vi "COD质控流程 (子VI).vi"(11 "COD":bool) -> (3 "布尔":bool)   [LabVIEW 2016, in "质控单元.lvlib"]
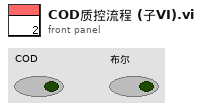
[diagram p1: front panel]
types:
  T1 = enum16{"待机", "启动水样测量", "水样测量中", "启动加标", "启动加标回收", "加标回收测量中", "结束"}
  T2 = cluster{"测量模式":enum16{"水样测量", "标样核查", "零点核查", "加标回收", "平行样", "校零", "校标"}}
  T3 = cluster{"量程":dbl, "检出限":dbl, "加标前水样浓度":dbl, "加标后水样浓度":dbl, "加标水杯定容体积":dbl, "加标母液浓度":dbl, "加标体积":dbl, "加标回收率":dbl}
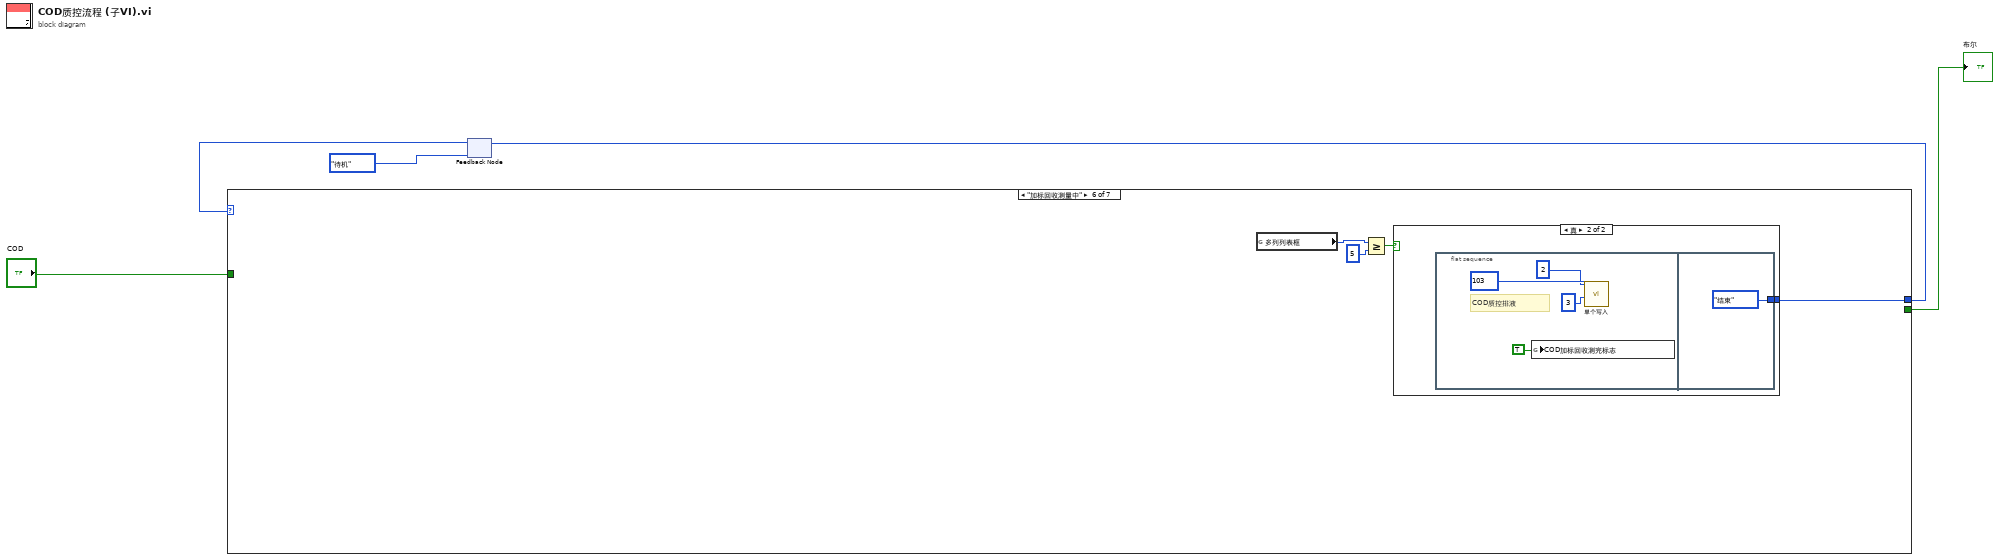
[diagram p0: block diagram]
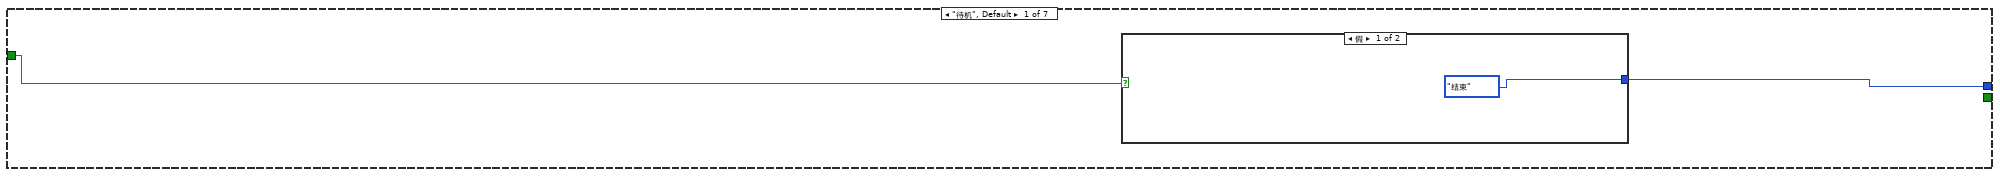
[diagram p2: hidden frame]
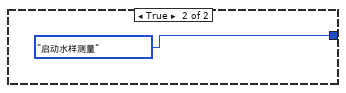
[diagram p3: hidden frame]
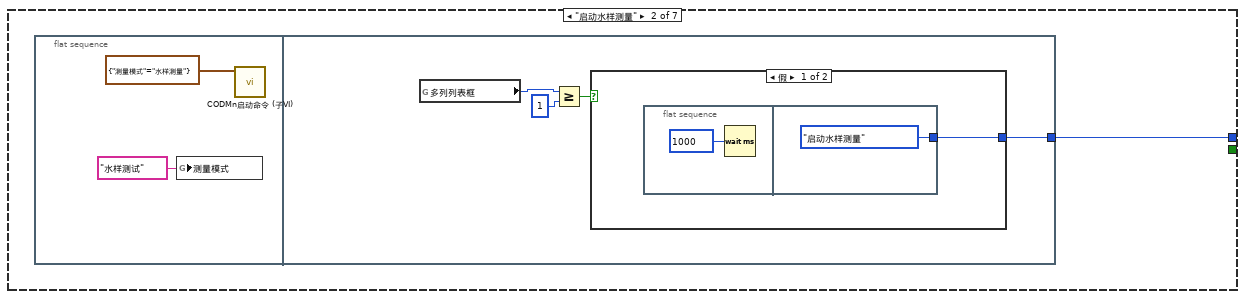
[diagram p4: hidden frame]
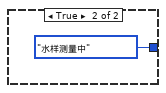
[diagram p5: hidden frame]
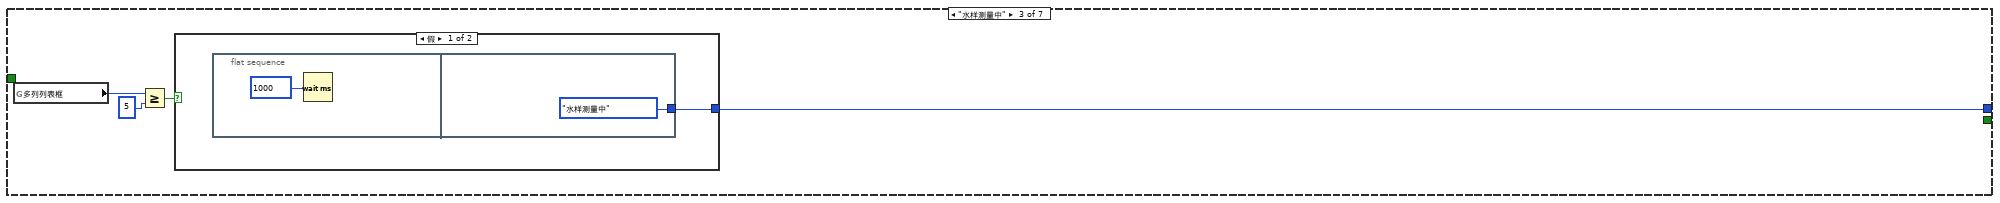
[diagram p6: hidden frame]
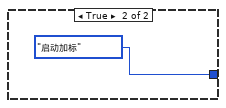
[diagram p7: hidden frame]
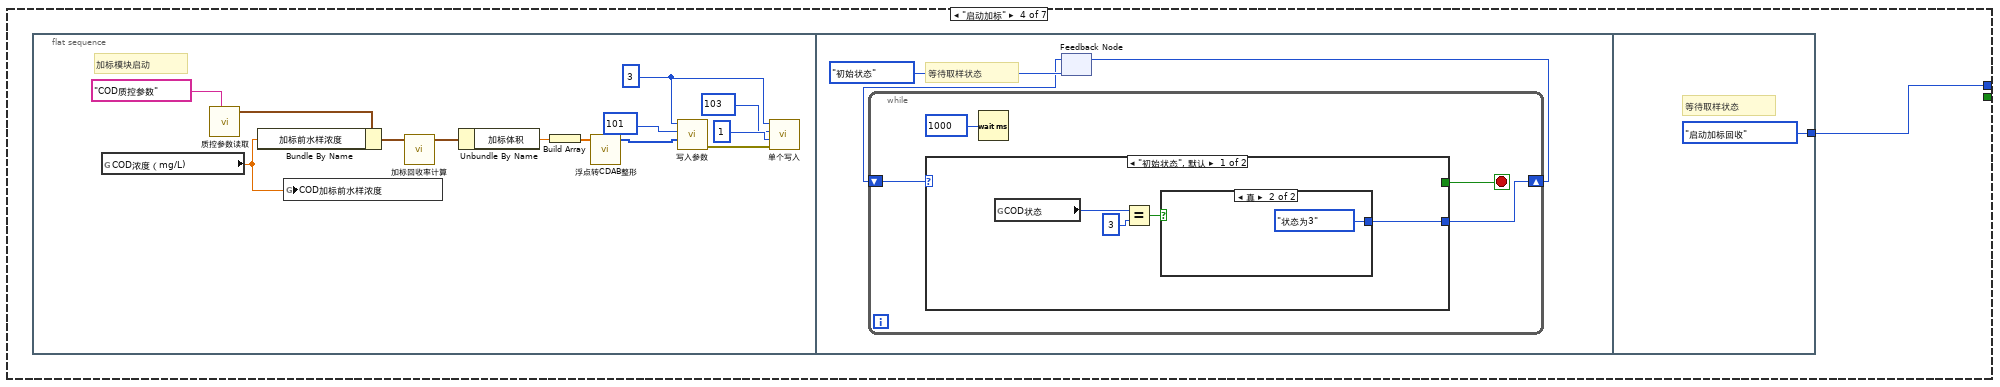
[diagram p8: hidden frame]
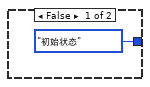
[diagram p9: hidden frame]
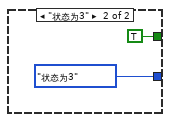
[diagram p10: hidden frame]
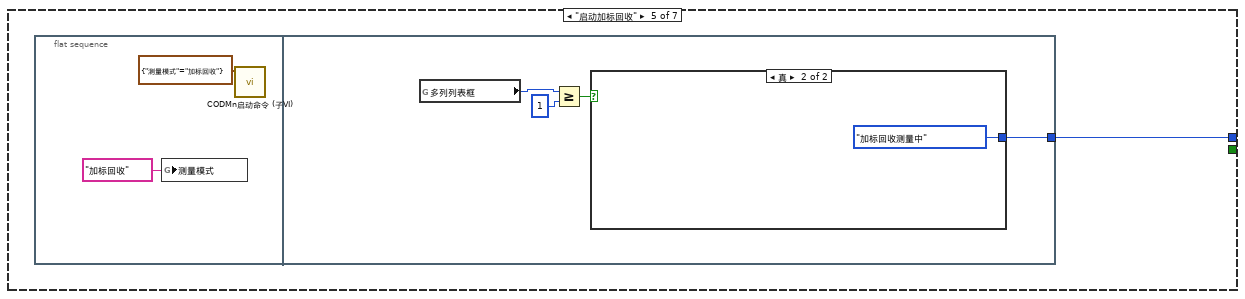
[diagram p11: hidden frame]
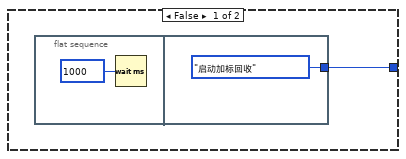
[diagram p12: hidden frame]
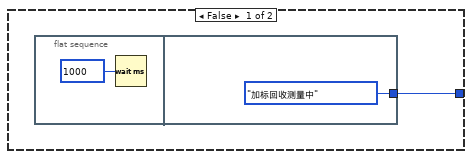
[diagram p13: hidden frame]
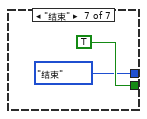
[diagram p14: hidden frame]
diagram:
  n1 = feedback #1(T1."待机") -> (w3:T1)
  n2 = case shown="\"加标回收测量中\"" w3 {
    tunnel: [w7 w10 w21 w29 w59 w70 T1."结束"] -> w4
    tunnel: [_ _ _ _ _ _ TRUE] -> w2
    tunnel: "COD" -> [w6 _ _ _ _ _ _]
    frame "待机", Default {
      n3 = case shown="假" w6 {
        tunnel: [T1."结束" T1."启动水样测量"] -> w7
        frame False {
        }
        frame True {
        }
      }
    }
    frame "启动水样测量" {
      n4 = flat-sequence {
        tunnel: [w13] -> w10
        frame #0 {
          n5 = global write "COD测量模式全局.vi" "测量模式"("水样测试" ("测量模式")) -> ()
          n6 = call "CODMn启动命令 (子VI).vi"("启动测量模式"=T2 {"测量模式"=enum."水样测量"}) -> ()  [unwired: 11 in]
        }
        frame #1 {
          n7 = global read "运行时序全局变量.vi" "多列列表框"() -> (w16:i32)
          n8 = Greater Or Equal?(x=w16, y=1) -> (x >= y?=w15:bool)
          n9 = case shown="假" w15 {
            tunnel: [w17 T1."水样测量中"] -> w13
            frame False {
              n10 = flat-sequence {
                tunnel: [T1."启动水样测量"] -> w17
                frame #0 {
                  n11 = Wait (ms)(milliseconds to wait=u32 1000 ("等待时间（毫秒）")) -> ()  [unwired: 1 out]
                }
                frame #1 {
                }
              }
            }
            frame True {
            }
          }
        }
      }
    }
    frame "水样测量中" {
      n12 = global read "运行时序全局变量.vi" "多列列表框"() -> (w22:i32)
      n13 = Greater Or Equal?(x=w22, y=5) -> (x >= y?=w23:bool)
      n14 = case shown="假" w23 {
        tunnel: [w25 T1."启动加标"] -> w21
        frame False {
          n15 = flat-sequence {
            tunnel: [T1."水样测量中"] -> w25
            frame #0 {
              n16 = Wait (ms)(milliseconds to wait=u32 1000 ("等待时间（毫秒）")) -> ()  [unwired: 1 out]
            }
            frame #1 {
            }
          }
        }
        frame True {
        }
      }
    }
    frame "启动加标" {
      n17 = flat-sequence {
        tunnel: [T1."启动加标回收"] -> w29
        frame #0 {
          w32 = u16 3 ("value")
          # "加标模块启动"
          n18 = global read "COD浓度全局变量.vi" "COD浓度（mg/L)"() -> (w30:dbl)
          n19 = call "质控参数读取.vi"("section"="COD质控参数") -> ("参数"=w40:T3)  [unwired: 9 in, 1 out]
          n20 = Bundle By Name(cluster=w40, "加标前水样浓度"=w30) -> (w41:T3)
          n21 = global write "水样浓度全局.vi" "COD加标前水样浓度"(w30) -> ()
          n22 = call "加标回收率计算.vi"("参数"=w41) -> ("参数 out"=w39:T3)  [unwired: 10 in]
          n23 = Unbundle By Name(w39) -> ("加标体积"=w31:dbl)
          n24 = Build Array(w31) -> (w38:dbl[])
          n25 = call "浮点转CDAB整形.vi"("浮点数"=w38) -> ("CDAB整形输出"=w33:u16[])  [unwired: 10 in]
          n26 = call "写入参数.vi"("values"=w33, "starting address"=u16 101, "Slave ID"=w32) -> ("error out"=w37:errorcluster)  [unwired: 8 in]
          n27 = call "单个写入.vi"("Error in"=w37, "value"=u16 1, "address"=u16 103, "Slave ID"=w32) -> ()  [unwired: 7 in, 1 out]
        }
        frame #1 {
          # "等待取样状态"
          n28 = feedback #2(enum16{"初始状态", "状态为3"}."初始状态") -> (w44:enum16{"初始状态", "状态为3"})
          n29 = while {
            shift-right: [w48] -> w43
            shift-left: w44 -> [w49]
            stop <- w47 stop-if-true
            n30 = case shown="\"初始状态\", 默认" w49 {
              tunnel: [w50 enum16{"初始状态", "状态为3"}."状态为3"] -> w48
              tunnel: [_ TRUE] -> w47
              frame "初始状态", Default {
                n31 = global read "氨氮加标回收状态全局变量.vi" "COD状态"() -> (w52:u16)
                n32 = Equal?(x=w52, y=u16 3) -> (x = y?=w51:bool)
                n33 = case shown="真" w51 {
                  tunnel: [enum16{"初始状态", "状态为3"}."初始状态" enum16{"初始状态", "状态为3"}."状态为3"] -> w50
                  frame False {
                  }
                  frame True {
                  }
                }
              }
              frame "状态为3" {
              }
            }
            n34 = Wait (ms)(milliseconds to wait=u32 1000 ("等待时间（毫秒）")) -> ()  [unwired: 1 out]
          }
          n35 = feedback-in #2(w43) -> ()
        }
        frame #2 {
          # "等待取样状态"
        }
      }
    }
    frame "启动加标回收" {
      n36 = flat-sequence {
        tunnel: [w62] -> w59
        frame #0 {
          n37 = global write "COD测量模式全局.vi" "测量模式"("加标回收" ("测量模式")) -> ()
          n38 = call "CODMn启动命令 (子VI).vi"("启动测量模式"=T2 {"测量模式"=enum."加标回收"}) -> ()  [unwired: 11 in]
        }
        frame #1 {
          n39 = global read "运行时序全局变量.vi" "多列列表框"() -> (w63:i32)
          n40 = Greater Or Equal?(x=w63, y=1) -> (x >= y?=w64:bool)
          n41 = case shown="真" w64 {
            tunnel: [w66 T1."加标回收测量中"] -> w62
            frame False {
              n42 = flat-sequence {
                tunnel: [T1."启动加标回收"] -> w66
                frame #0 {
                  n43 = Wait (ms)(milliseconds to wait=u32 1000 ("等待时间（毫秒）")) -> ()  [unwired: 1 out]
                }
                frame #1 {
                }
              }
            }
            frame True {
            }
          }
        }
      }
    }
    frame "加标回收测量中" {
      n44 = global read "运行时序全局变量.vi" "多列列表框"() -> (w71:i32)
      n45 = Greater Or Equal?(x=w71, y=5) -> (x >= y?=w72:bool)
      n46 = case shown="真" w72 {
        tunnel: [w74 w77] -> w70
        frame False {
          n47 = flat-sequence {
            tunnel: [T1."加标回收测量中"] -> w74
            frame #0 {
              n48 = Wait (ms)(milliseconds to wait=u32 1000 ("等待时间（毫秒）")) -> ()  [unwired: 1 out]
            }
            frame #1 {
            }
          }
        }
        frame True {
          n49 = flat-sequence {
            tunnel: [T1."结束"] -> w77
            frame #0 {
              # "COD质控排液"
              n50 = global write "质控测完标志全局 1.vi" "COD加标回收测完标志"(TRUE ("COD加标回收测完标志")) -> ()
              n51 = call "单个写入.vi"("value"=u16 3, "address"=u16 103, "Slave ID"=u8 2) -> ()  [unwired: 8 in, 1 out]
            }
            frame #1 {
            }
          }
        }
      }
    }
    frame "结束" {
    }
  }
  "布尔" <- w2
  n52 = feedback-in #1(w4) -> ()
